vi "Flappy_main.vi"() -> ()   [LabVIEW 8.6]
uses:
  <vilib>/Utility/miscctls.llb/LVPositionTypeDef.ctl
  <vilib>/Utility/inputDevices.llb/keyboardAcquire.vi
  <vilib>/Utility/inputDevices.llb/closeKeyboard.vi
panel:
  in  "QRCode":bool
  in  "obs_air":bool
  out "Score":i32
  out "BG_ref":refnum<vi>[](array[refnum])
  out "ball":bool
  in  "Mov_Spd":i32
  in  "g":dbl
  out "Slide_scr":u8(slide)
  in  "L_limit":bool
  out "Gmsg":string
  out "Obs_D_ref":refnum<vi>[](array[refnum])
  out "Obs_U_ref":refnum<vi>[](array[refnum])
  in  "obsU 5":bool
  in  "obsD 5":bool
  in  "obsU 4":bool
  in  "obsD 4":bool
  in  "obsD 3":bool
  in  "obsU 2":bool
  in  "obsD 2":bool
  in  "obsU 1":bool
  in  "obsD 1":bool
  in  "start":bool
  in  "obsU 3":bool
  # "by hls.ding@gmail."
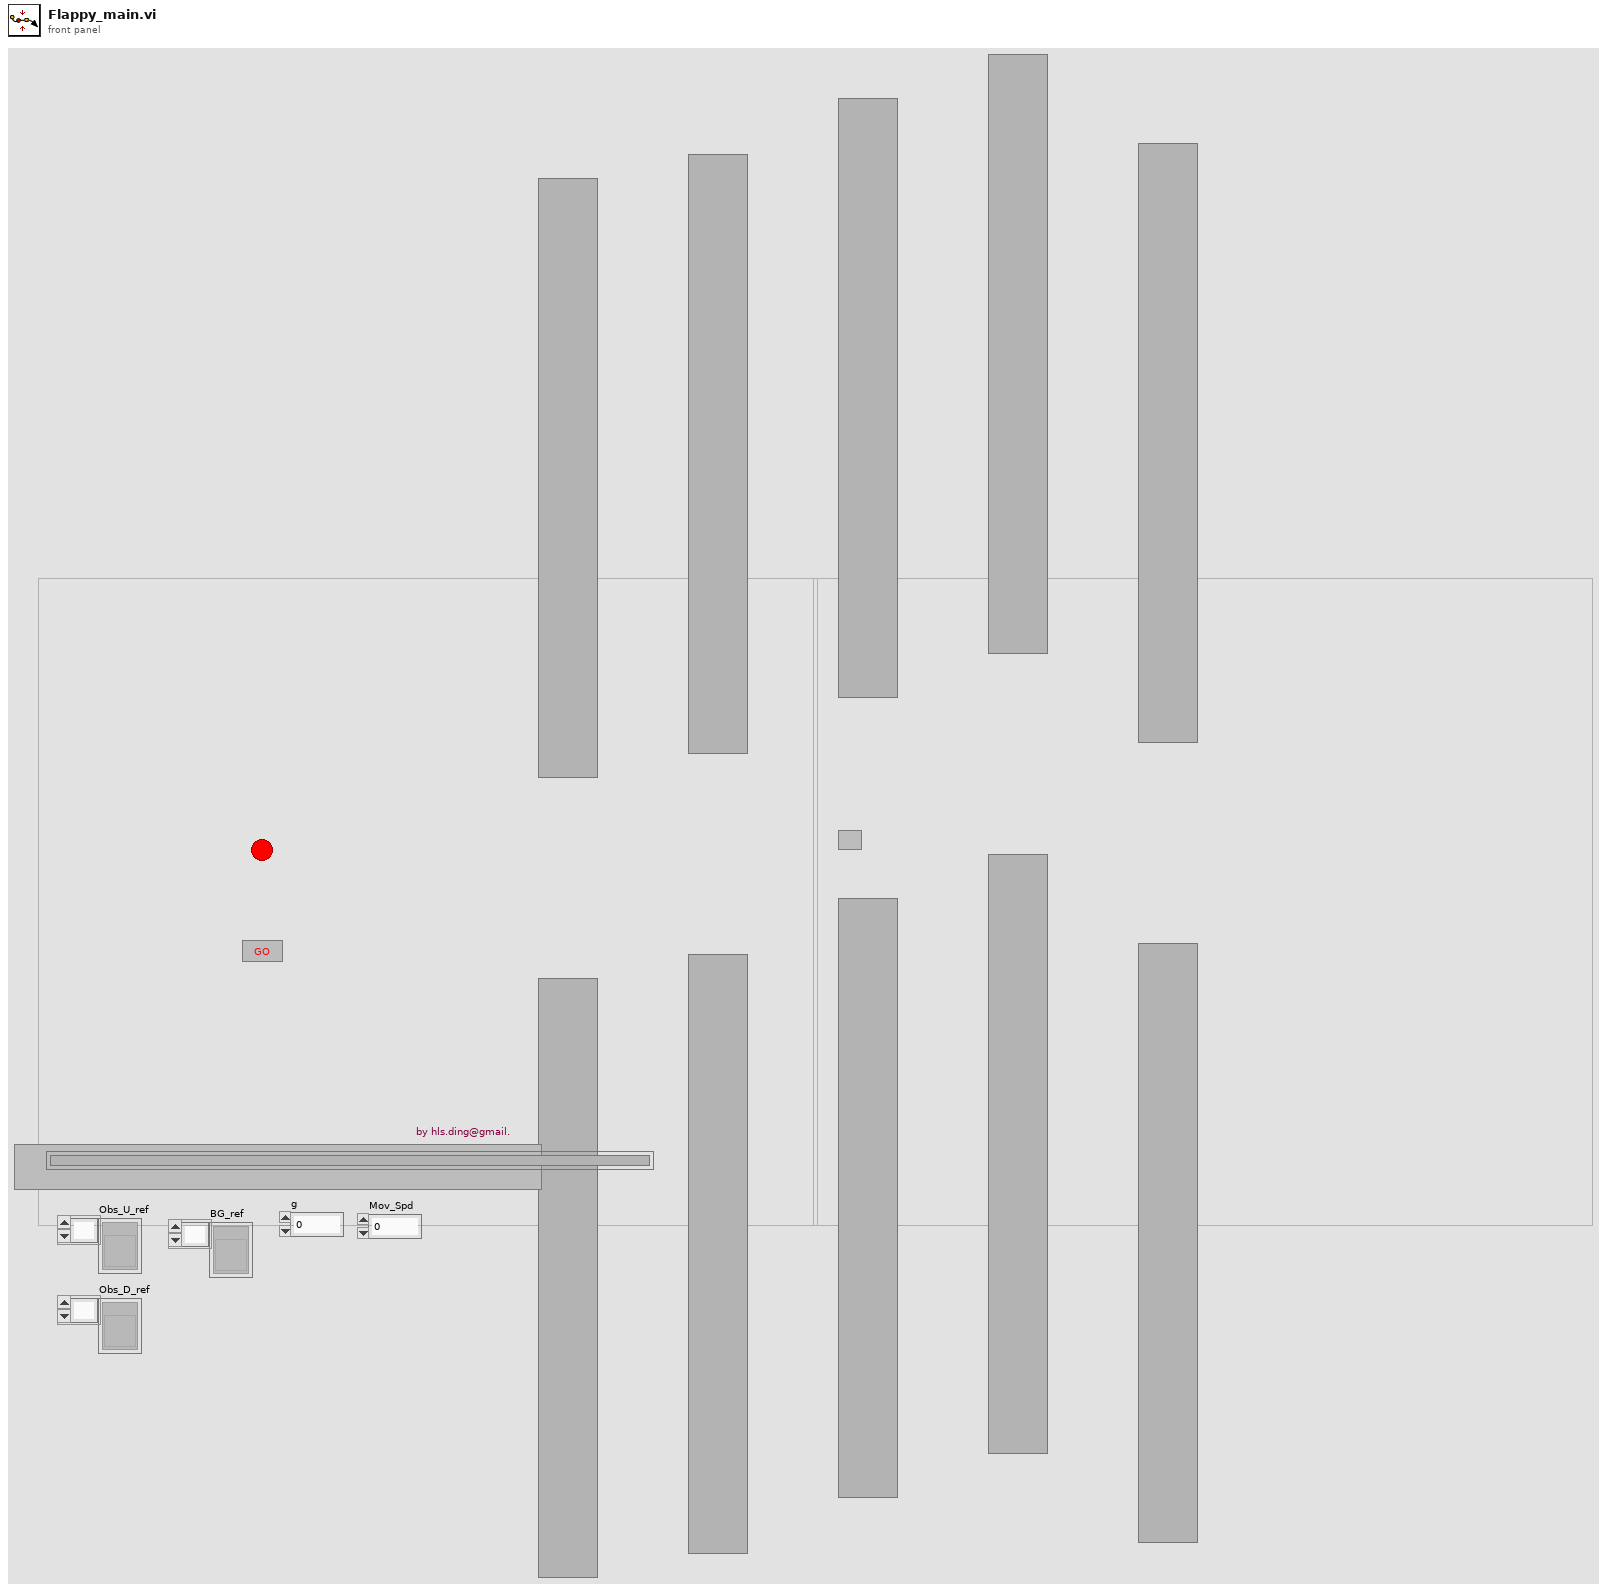
[diagram p1: front panel]
types:
  T1 = typedef "LVPositionTypeDef.ctl" = cluster{"Left":i32, "Top":i32}
  T2 = enum16{"0", "1", "2", "3", "4", "5", "6", "7", "8", "9", "A", "B", "C", "D", "E", "F", "G", "H", "I", "J", "K", "L", "M", "N", "O", "P", "Q", "R", "S", "T", "U", "V", "W", "X", "Y", "Z", "F1", "F2", "F3", "F4", "F5", "F6", "F7", "F8", "F9", "F10", "F11", "F12", "F13", "F14", "F15", "ADD", "BACK", "BACKSLASH", "CAPITAL", "COMMA", "DECIMAL", "DELETE", "DIVIDE", "DOWN", "END", "EQUALS", "ESCAPE", "GRAVE (`)", "HOME", "INSERT", "LBRACKET", "LCONTROL", "LEFT", "L ALT", "LSHIFT", "LWIN", "MINUS", "MULTIPLY", "NEXT", "NUMLOCK", "NUMPAD_0", "NUMPAD_1", "NUMPAD_2", "NUMPAD_3", "NUMPAD_4", "NUMPAD_5", "NUMPAD_6", "NUMPAD_7", "NUMPAD_8", "NUMPAD_9", "PAUSE", "PERIOD", "PRIOR (PG UP)", "RBRACKET", "RCONTROL", "RETURN", "RIGHT", "R ALT", "RSHIFT", "RWIN", "SCROLL", "SEMICOLON", "SLASH", "SPACE", "SUBTRACT", "TAB", "UP", "ENTER (num pad)", "' (quote)"}
  T3 = enum16{"0", "1", "2", "3", "4", "5", "6", "7", "8", "9", "A", "B", "C", "D", "E", "F", "G", "H", "I", "J", "K", "L", "M", "N", "O", "P", "Q", "R", "S", "T", "U", "V", "W", "X", "Y", "Z", "F1", "F2", "F3", "F4", "F5", "F6", "F7", "F8", "F9", "F10", "F11", "F12", "F13", "F14", "F15", "ADD", "BACK", "BACKSLASH", "CAPITAL", "COMMA", "DECIMAL", "DELETE", "DIVIDE", "DOWN", "END", "EQUALS", "ESCAPE", "GRAVE (`)", "HOME", "INSERT", "LBRACKET", "LCONTROL", "LEFT", "L ALT", "LSHIFT", "LWIN", "MINUS", "MULTIPLY", "NEXT", "NUMLOCK", "NUMPAD_0", "NUMPAD_1", "NUMPAD_2", "NUMPAD_3", "NUMPAD_4", "NUMPAD_5", "NUMPAD_6", "NUMPAD_7", "NUMPAD_8", "NUMPAD_9", "PAUSE", "PERIOD", "PRIOR (PG UP)", "RBRACKET", "RCONTROL", "RETURN", "RIGHT", "R ALT", "RSHIFT", "RWIN", "SCROLL", "SEMICOLON", "SLASH", "SPACE", "SUBTRACT", "TAB", "UP", "ENTER (num pad)", "' (quote)"}[]
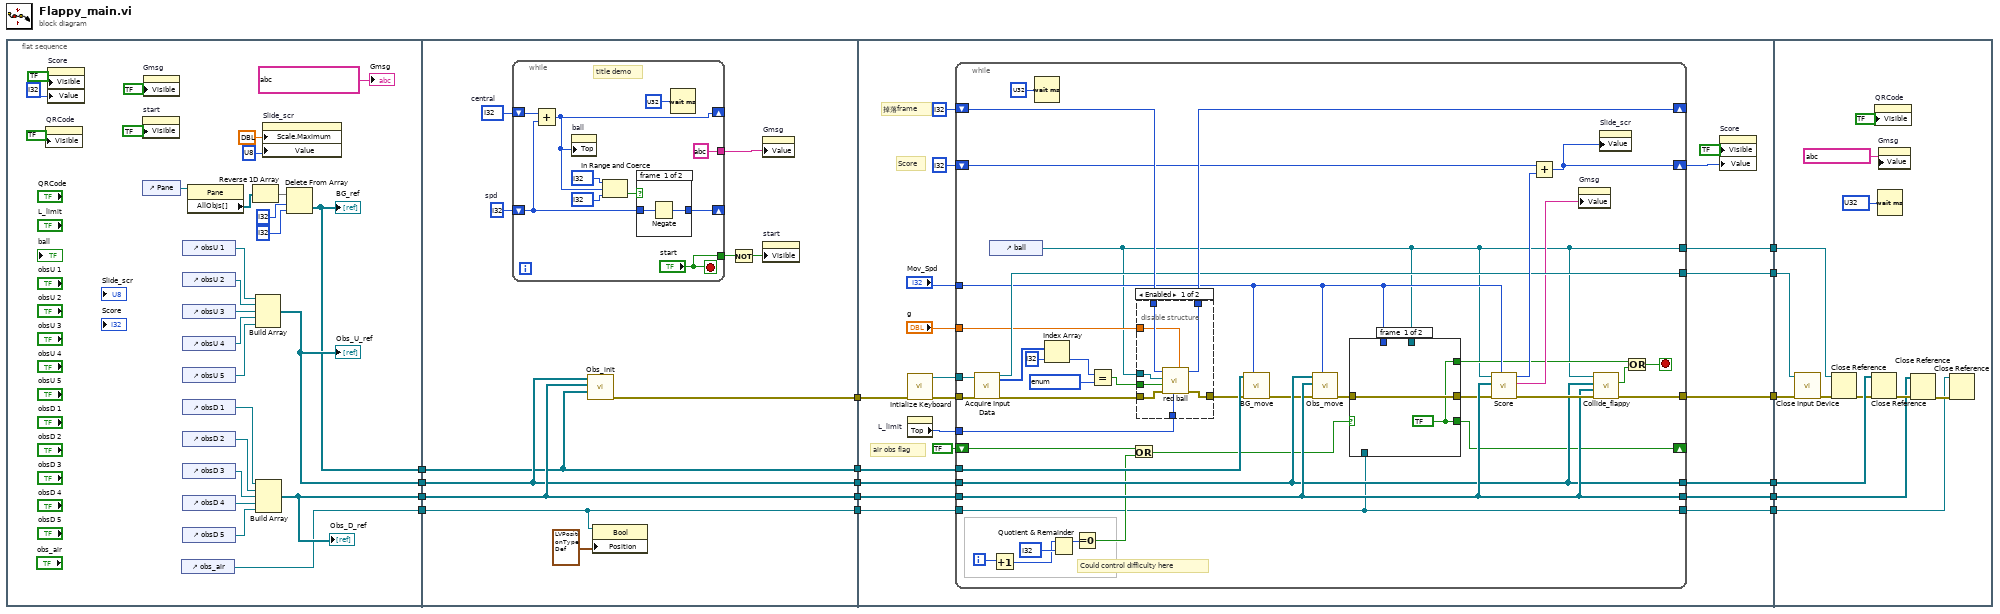
[diagram p0: block diagram]
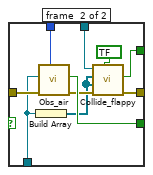
[diagram p3: hidden frame]
diagram:
  n1 = flat-sequence {
    tunnel: [w30] -> w13
    tunnel: [w29] -> w12
    tunnel: [w19] -> w4
    tunnel: [w18] -> w3
    tunnel: w13 -> [w48]
    tunnel: w12 -> [w47]
    tunnel: [w49] -> w8
    tunnel: [w48] -> w7
    tunnel: [w47] -> w6
    tunnel: [w46] -> w5
    tunnel: w4 -> [w46]
    tunnel: w3 -> [w43]
    tunnel: [w43] -> w2
    tunnel: [w82] -> w15
    tunnel: [w81] -> w14
    tunnel: [w76] -> w11
    tunnel: [w75] -> w10
    tunnel: [w74] -> w9
    tunnel: w8 -> [w73]
    tunnel: w7 -> [w72]
    tunnel: w6 -> [w71]
    tunnel: w5 -> [w70]
    tunnel: w2 -> [w69]
    tunnel: [w67] -> w1
    tunnel: w15 -> [w162]
    tunnel: w14 -> [w161]
    tunnel: w11 -> [w159]
    tunnel: w10 -> [w158]
    tunnel: w9 -> [w157]
    tunnel: w1 -> [w152]
    frame #0 {
      n2 = property on="QRCode" class="Bool (strict)"("Visible"=bool ?) -> ()  [unwired: 2 in, 2 out]
      n3 = property on="Score" class="DigNum (strict)"("Visible"=bool ?, "Value"=i32 ? ("Score")) -> ()  [unwired: 2 in, 2 out]
      n4 = property on="start" class="Bool"("Visible"=bool ?) -> ()  [unwired: 2 in, 2 out]
      n5 = control-ref of="Pane"() -> (w22:refnum<vi>)
      n6 = property on="Gmsg" class="Str"("Visible"=bool ?) -> ()  [unwired: 2 in, 2 out]
      n7 = control-ref of="obs_air"() -> (w18:refnum<vi>)
      n8 = control-ref of="obsU 1"() -> (w42:refnum<vi>)
      n9 = control-ref of="obsU 2"() -> (w41:refnum<vi>)
      n10 = control-ref of="obsU 3"() -> (w40:refnum<vi>)
      n11 = control-ref of="obsU 4"() -> (w39:refnum<vi>)
      n12 = control-ref of="obsU 5"() -> (w38:refnum<vi>)
      n13 = control-ref of="obsD 1"() -> (w37:refnum<vi>)
      n14 = control-ref of="obsD 2"() -> (w36:refnum<vi>)
      n15 = control-ref of="obsD 3"() -> (w35:refnum<vi>)
      n16 = control-ref of="obsD 4"() -> (w34:refnum<vi>)
      n17 = control-ref of="obsD 5"() -> (w33:refnum<vi>)
      n18 = property class="Pane"(reference=w22) -> ("AllObjs[]"=w24:refnum<vi>[])  [unwired: 1 in, 2 out]
      n19 = Reverse 1D Array(array=w24) -> (reversed array=w23:refnum<vi>[])
      n20 = Build Array(w42, w41, w40, w39, w38) -> (w29:refnum<vi>[])
      "Obs_U_ref" <- w29
      n21 = Build Array(w37, w36, w35, w34, w33) -> (w30:refnum<vi>[])
      "Obs_D_ref" <- w30
      n22 = property on="Slide_scr" class="Slide (strict)"("Scale.Maximum"=dbl ? ("Scale.Range:Maximum"), "Value"=u8 ? ("Slide_scr")) -> ()  [unwired: 2 in, 2 out]
      n23 = Delete From Array(array=w23, length=i32 ? ("index"), index=i32 ?) -> (deleted portion=w19:refnum<vi>[])  [unwired: 1 out]
      "BG_ref" <- w19
      "Gmsg" <- string ? ("Gmsg")
    }
    frame #1 {
      w52 = i32 ?  # spd
      w53 = i32 ?  # central
      n24 = while {
        shift-right: [w56] -> _
        shift-left: w53 -> [w63]
        shift-right: [w58] -> _
        shift-left: w52 -> [w60]
        tunnel: ["start"] -> w51
        tunnel: [string ? ("Gmsg")] -> w45
        stop <- "start" stop-if-true
        # "title demo"
        n25 = Add(x=w63, y=w60) -> (x+y=w56:i32)
        n26 = property on="ball" class="Bool (strict)"("Top"=w56) -> ()  [unwired: 2 in, 2 out]
        n27 = In Range and Coerce(upper limit=i32 ?, x=w56, lower limit=i32 ?) -> (In Range?=w59:bool)  [unwired: 1 out]
        n28 = case shown="True" w59 {
          tunnel: w60 -> [w65 w66]
          tunnel: [w64 w66] -> w58
          frame #0 {
            n29 = Negate(x=w65) -> (-x=w64:i32)
          }
          frame #1 {
          }
        }
        n30 = Wait (ms)(milliseconds to wait=u32 ?) -> ()  [unwired: 1 out]
      }
      n31 = call "Obs_init.vi"("BG_ref"=w46, "ObsD_in"=w48, "ObsU_in"=w47) -> ("error IO"=w49:errorcluster)  [unwired: 8 in]
      n32 = property class="Bool"(reference=w43, "Position"=T1 ?) -> ()  [unwired: 1 in, 2 out]
      n33 = Not(x=w51) -> (.not. x?=w50:bool)
      n34 = property on="Gmsg" class="Str"("Value"=w45) -> ()  [unwired: 2 in, 2 out]
      n35 = property on="start" class="Bool"("Visible"=w50) -> ()  [unwired: 2 in, 2 out]
    }
    frame #2 {
      # "air obs flag"
      # "Score"
      # "掉落frame"
      n36 = call <vilib>:"Intialize Keyboard.vi"("error in (no error)"=w73) -> ("error out"=w86:errorcluster, "device ID"=w87:refnum<k1>)  [unwired: 9 in]
      n37 = property on="L_limit" class="Bool"() -> ("Top"=w84:i32)  [unwired: 2 in, 2 out]
      n38 = while {
        tunnel: w87 -> [w128]
        tunnel: w86 -> [w127]
        shift-right: [w124] -> _
        shift-left: i32 ? ("index") -> [w121]
        tunnel: w84 -> [w123]
        shift-right: [w110] -> w80
        shift-left: i32 ? -> [w119]
        tunnel: [w111] -> w81
        tunnel: [w115] -> w82
        tunnel: "g" -> [w114]
        tunnel: "Mov_Spd" -> [w93]
        tunnel: [w108] -> w76
        tunnel: [w109] -> w75
        tunnel: [w89] -> w74
        tunnel: w72 -> [w109]
        tunnel: w71 -> [w108]
        tunnel: w70 -> [w106]
        tunnel: w69 -> [w88]
        shift-right: [w99] -> _
        shift-left: bool ? -> [w101]
        tunnel: [w88] -> w67
        i -> [w98]
        stop <- w92 stop-if-true
        # "Could control difficulty here"
        n39 = call-poly <vilib>:"Acquire Input Data.vi"("device ID"=w128, "error in (no error)"=w127) -> ("device ID"=w115:refnum<k1>, "keys pressed"=w126:T3, "error out"=w120:errorcluster)  [unwired: 15 in]
        n40 = control-ref of="ball"() -> (w89:refnum<vi>)
        n41 = Increment(x=w98) -> (x+1=w97:i32)
        n42 = Wait (ms)(milliseconds to wait=u32 ?) -> ()  [unwired: 1 out]
        n43 = Index Array(array=w126, index=i32 ?) -> (element=w116:T2)
        n44 = Quotient & Remainder(x=w97, y=i32 ?) -> (x-y*floor(x/y)=w103:i32)  [unwired: 1 out]
        n45 = Equal To 0?(x=w103) -> (x = 0?=w102:bool)
        n46 = Equal?(x=w116, y=T2 ? ("keyType 3")) -> (x = y?=w113:bool)
        n47 = Or(x=w101, y=w102) -> (x .or. y?=w100:bool)
        n48 = disable-structure shown="Enabled" {
          disable-tunnel: [w148 _] -> w124
          disable-tunnel: w123 -> [w147 _]
          disable-tunnel: w121 -> [w146 _]
          disable-tunnel: [w145 w149] -> w96
          disable-tunnel: w120 -> [w144 w149]
          disable-tunnel: w89 -> [w143 _]
          disable-tunnel: w114 -> [w142 _]
          disable-tunnel: w113 -> [w141 _]
          frame #0 {
            n49 = call "red ball.vi"("g"=w142, "L_limit"=w147, "error in"=w144, "Jump"=w141, "Red_ball"=w143, "frame in"=w146) -> ("error out"=w145:errorcluster, "frame out"=w148:i32)  [unwired: 4 in]
          }
          frame #1 {
          }
        }
        n50 = call "BG_move.vi"("Mov_Spd"=w93, "error in"=w96, "BG_ref"=w106) -> ("error out"=w107:errorcluster)  [unwired: 8 in]
        n51 = call "Obs_move.vi"("Mov_Spd"=w93, "error in"=w107, "Obst D_REF"=w109, "Obst U_Ref"=w108) -> ("error out"=w95:errorcluster)  [unwired: 7 in]
        n52 = case shown="True" w100 {
          tunnel: w95 -> [w130 w140]
          tunnel: [w130 w136] -> w94
          tunnel: [w129 w139] -> w99
          tunnel: w88 -> [_ w133]
          tunnel: w93 -> [_ w138]
          tunnel: [w129 w135] -> w90
          tunnel: w89 -> [_ w131]
          frame #0 {
            w129 = bool ? ("active")
          }
          frame #1 {
            n53 = Build Array(w133) -> (w132:refnum<vi>[])
            n54 = call "Obs_air.vi"("Mov_Spd"=w138, "error in"=w140, "Obs A_Ref"=w133) -> ("error out"=w137:errorcluster, "active"=w139:bool)  [unwired: 7 in]
            n55 = call "Collide_flappy.vi"("obs_a?"=bool ?, "error in"=w137, "Obs D_in"=w132, "Obs U_in"=w132, "ball in"=w131) -> ("error Out"=w136:errorcluster, "bump"=w135:bool)  [unwired: 5 in]
          }
        }
        n56 = call "Score.vi"("Mov_Spd"=w93, "error in"=w94, "Obs D_in"=w109, "Ball in"=w89) -> ("error out"=w112:errorcluster, "Msg"=w105:string, "Add"=w118:i32)  [unwired: 5 in]
        n57 = Add(x=w119, y=w118) -> (x+y=w110:i32)
        n58 = property on="Gmsg" class="Str"("Value"=w105) -> ()  [unwired: 2 in, 2 out]
        n59 = call "Collide_flappy.vi"("error in"=w112, "Obs D_in"=w109, "Obs U_in"=w108, "ball in"=w89) -> ("error Out"=w111:errorcluster, "bump"=w91:bool)  [unwired: 6 in]
        n60 = property on="Slide_scr" class="Slide (strict)"("Value"=w110) -> ()  [unwired: 2 in, 2 out]
        n61 = Or(x=w90, y=w91) -> (x .or. y?=w92:bool)
      }
      n62 = property on="Score" class="DigNum (strict)"("Visible"=bool ?, "Value"=w80) -> ()  [unwired: 2 in, 2 out]
    }
    frame #3 {
      n63 = call-poly <vilib>:"Close Input Device.vi"("error in (no error)"=w161, "device ID"=w162) -> ("error out"=w156:errorcluster)  [unwired: 8 in]
      n64 = Close Reference(reference=w157, error in (no error)=w156) -> (error out=w155:errorcluster)
      n65 = Close Reference(reference=w159, error in (no error)=w155) -> (error out=w160:errorcluster)
      n66 = property on="QRCode" class="Bool (strict)"("Visible"=bool ?) -> ()  [unwired: 2 in, 2 out]
      n67 = Wait (ms)(milliseconds to wait=u32 ?) -> ()  [unwired: 1 out]
      n68 = property on="Gmsg" class="Str"("Value"=string ? ("Gmsg")) -> ()  [unwired: 2 in, 2 out]
      n69 = Close Reference(reference=w158, error in (no error)=w160) -> (error out=w153:errorcluster)
      n70 = Close Reference(reference=w152, error in (no error)=w153) -> ()  [unwired: 1 out]
    }
  }
